vi "Write Boolean.vi"(8 "error in (no error)":errorcluster, 10 "Boolean":bool, 11 "Set Boolean in":refnum<class "Set Boolean.lvclass">) -> (0 "error out":errorcluster, 3 "Set Boolean out":refnum<class "Set Boolean.lvclass">)   [LabVIEW 2021, in "BT.lvlib" / "Set Boolean.lvclass"]
uses:
  Set Boolean.lvclass
  Set Boolean.lvclass/Set Boolean.ctl
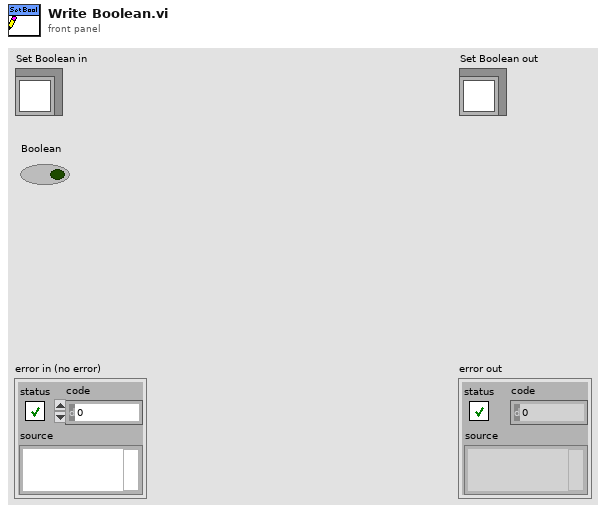
[diagram p1: front panel]
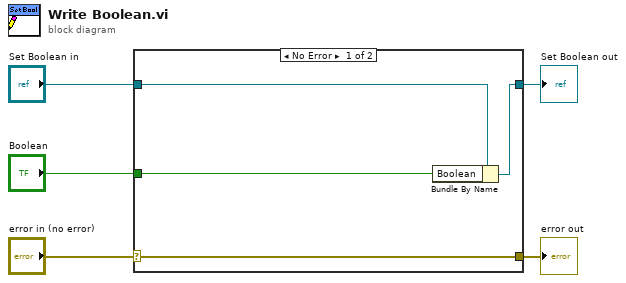
[diagram p0: block diagram]
diagram:
  n1 = case shown="No Error" "error in (no error)" {
    selector: "error in (no error)" -> [w9 w10]
    tunnel: [w9 w10] -> w4
    tunnel: [w7 w11] -> w2
    tunnel: "Set Boolean in" -> [w8 w11]
    tunnel: "Boolean" -> [w6 _]
    frame No Error {
      n2 = Bundle By Name(cluster=w8, "Boolean"=w6) -> (w7:refnum<class "Set Boolean.lvclass">)
    }
    frame Error {
    }
  }
  "error out" <- w4
  "Set Boolean out" <- w2
